vi "MakeCommandUnique.vi"(8 "error in (no error)":errorcluster, 11 "Command":string) -> (0 "error out":errorcluster, 3 "Unique Command":string)   [LabVIEW 2019]
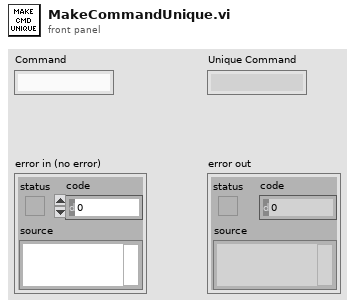
[diagram p1: front panel]
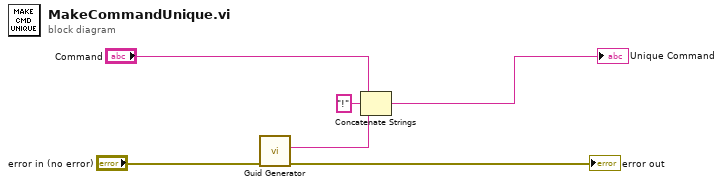
[diagram p0: block diagram]
diagram:
  n1 = call <vilib>:"Guid Generator.vi"("error in (no error)"="error in (no error)") -> ("error out"=→"error out":errorcluster, "GUID"=w2:string)  [unwired: 9 in]
  n2 = Concatenate Strings("Command", "!" ("string"), w2) -> (→"Unique Command":string)
